vi "Convert Point to Coord.vi"(8 "error in":errorcluster, 10 "Overlay":T1={"Name"="p0", "Data"={"Points"=array[7388 elements], "Voltages"=array[7388 elements]}}, 11 "BigMAQ in":refnum<class "BigMAQ.lvclass">) -> (0 "error out":errorcluster, 1 "Voltage Constant?":bool, 2 "output cluster":T1, 3 "BigMAQ out":refnum<class "BigMAQ.lvclass">)   [LabVIEW 2019, in "BigMAQ.lvclass"]
uses:
  BigMAQ.lvclass
  Overlay.ctl
  BigMAQ.lvclass/BigMAQ.ctl
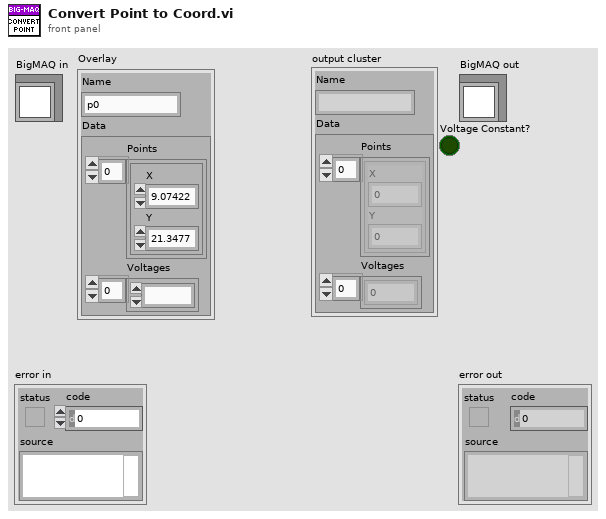
[diagram p1: front panel]
types:
  T1 = typedef "BigMAQ.lvclass/Overlay.ctl" = cluster{"Name":string, "Data":cluster{"Points":cluster{"X":dbl, "Y":dbl}[], "Voltages":dbl[]}}
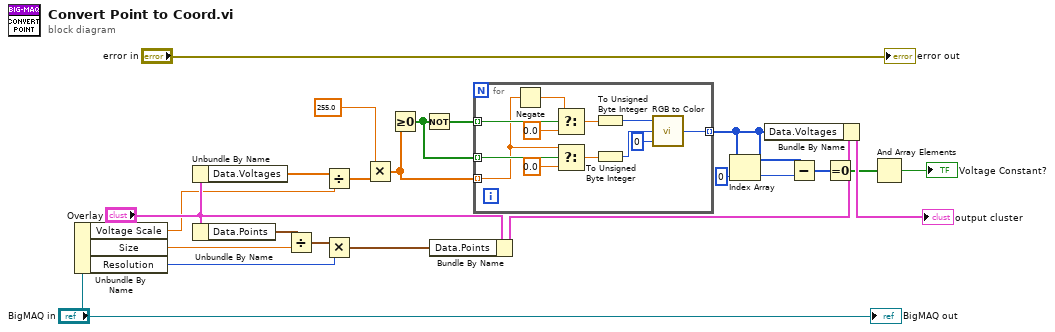
[diagram p0: block diagram]
diagram:
  n1 = Unbundle By Name("BigMAQ in") -> ("Voltage Scale"=w1:dbl, "Size"=w3:dbl, "Resolution"=w2:i32)
  n2 = Unbundle By Name("Overlay") -> ("Data.Voltages"=w19:dbl[])
  n3 = Unbundle By Name("Overlay") -> ("Data.Points"=w22:cluster{"X":dbl, "Y":dbl}[])
  n4 = Divide(x=w22, y=w3) -> (x/y=w21:cluster{"X":dbl, "Y":dbl}[])
  n5 = Divide(x=w19, y=w1) -> (x/y=w18:dbl[])
  n6 = Multiply(x=w21, y=w2) -> (x*y=w20:cluster{"X":dbl, "Y":dbl}[])
  n7 = Multiply(x=255.0, y=w18) -> (x*y=w17:dbl[])
  n8 = Greater Or Equal To 0?(x=w17) -> (x >= 0?=w14:bool[])
  n9 = Not(x=w14) -> (.not. x?=w15:bool[])
  n10 = Bundle By Name(cluster="Overlay", "Data.Points"=w20) -> (w13:T1)
  n11 = for {
    tunnel: w15 -> [w35] mode=indexing
    tunnel: w17 -> [w28] mode=indexing
    tunnel: w14 -> [w29] mode=indexing
    tunnel: [w24] -> w10 mode=indexing
    n12 = Negate(x=w28) -> (-x=w31:dbl)
    n13 = Select(t=w31, s=w35, f=0.0) -> (s? t:f=w34:dbl)
    n14 = Select(t=w28, s=w29, f=0.0) -> (s? t:f=w27:dbl)
    n15 = To Unsigned Byte Integer(number=w34) -> (unsigned 8bit integer=w33:u8)
    n16 = To Unsigned Byte Integer(number=w27) -> (unsigned 8bit integer=w26:u8)
    n17 = call <vilib>:"RGB to Color.vi"("B"=u8 0, "G"=w26, "R"=w33) -> ("Color"=w24:u32)
  }
  n18 = Index Array(array=w10, index=0) -> (element=w9:u32)
  n19 = Bundle By Name(cluster=w13, "Data.Voltages"=w10) -> (→"output cluster":T1)
  n20 = Subtract(x=w10, y=w9) -> (x-y=w8:u32[])
  n21 = Equal To 0?(x=w8) -> (x = 0?=w7:bool[])
  n22 = And Array Elements(Boolean array=w7) -> (logical AND=→"Voltage Constant?":bool)
  "error out" <- "error in"
  "BigMAQ out" <- "BigMAQ in"
